vi "ApproachMonitor.vi"() -> ()   [LabVIEW 2021]
uses:
  <userlib>/Nanonis Prog Interface V5/Nanonis Prog Interface.lvlib
panel:
  in  "Walker Frequency (Hz)":dbl=220.0
  in  "Bias (V)":dbl=-1.2 format="%#_6p"
  in  "Walker voltage (V)":dbl=220.0
  in  "Time between checks (ms)":i32=20000
  in  "Averages":i32=50
  in  "milliseconds to wait":u32=1000
  out "Delta":cluster{i32, sgl}[](graph)
  out "Capacitance":cluster{i32, sgl}[](graph)
  # "MAKE SURE FAST APPROACH IS NOT TURNED ON!!!!!!!!!!"
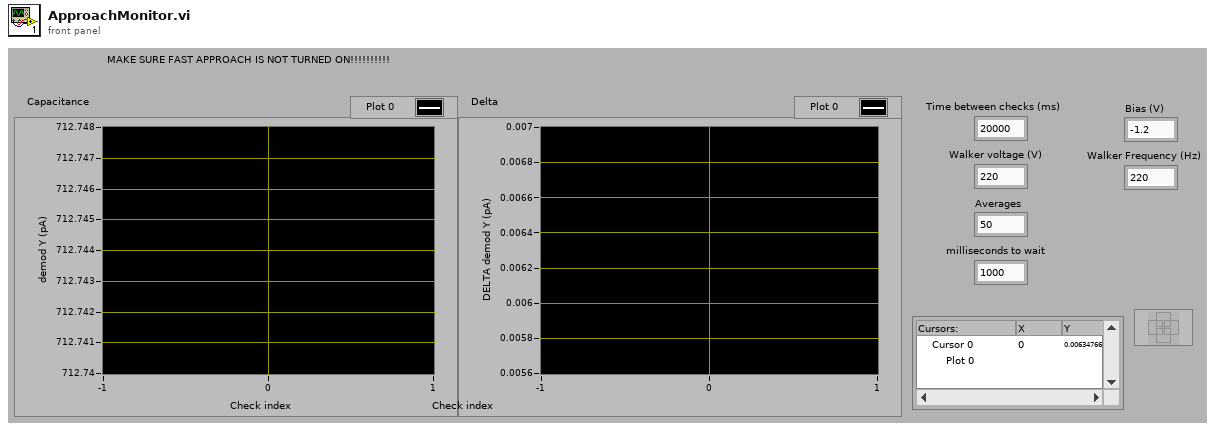
[diagram p1: front panel]
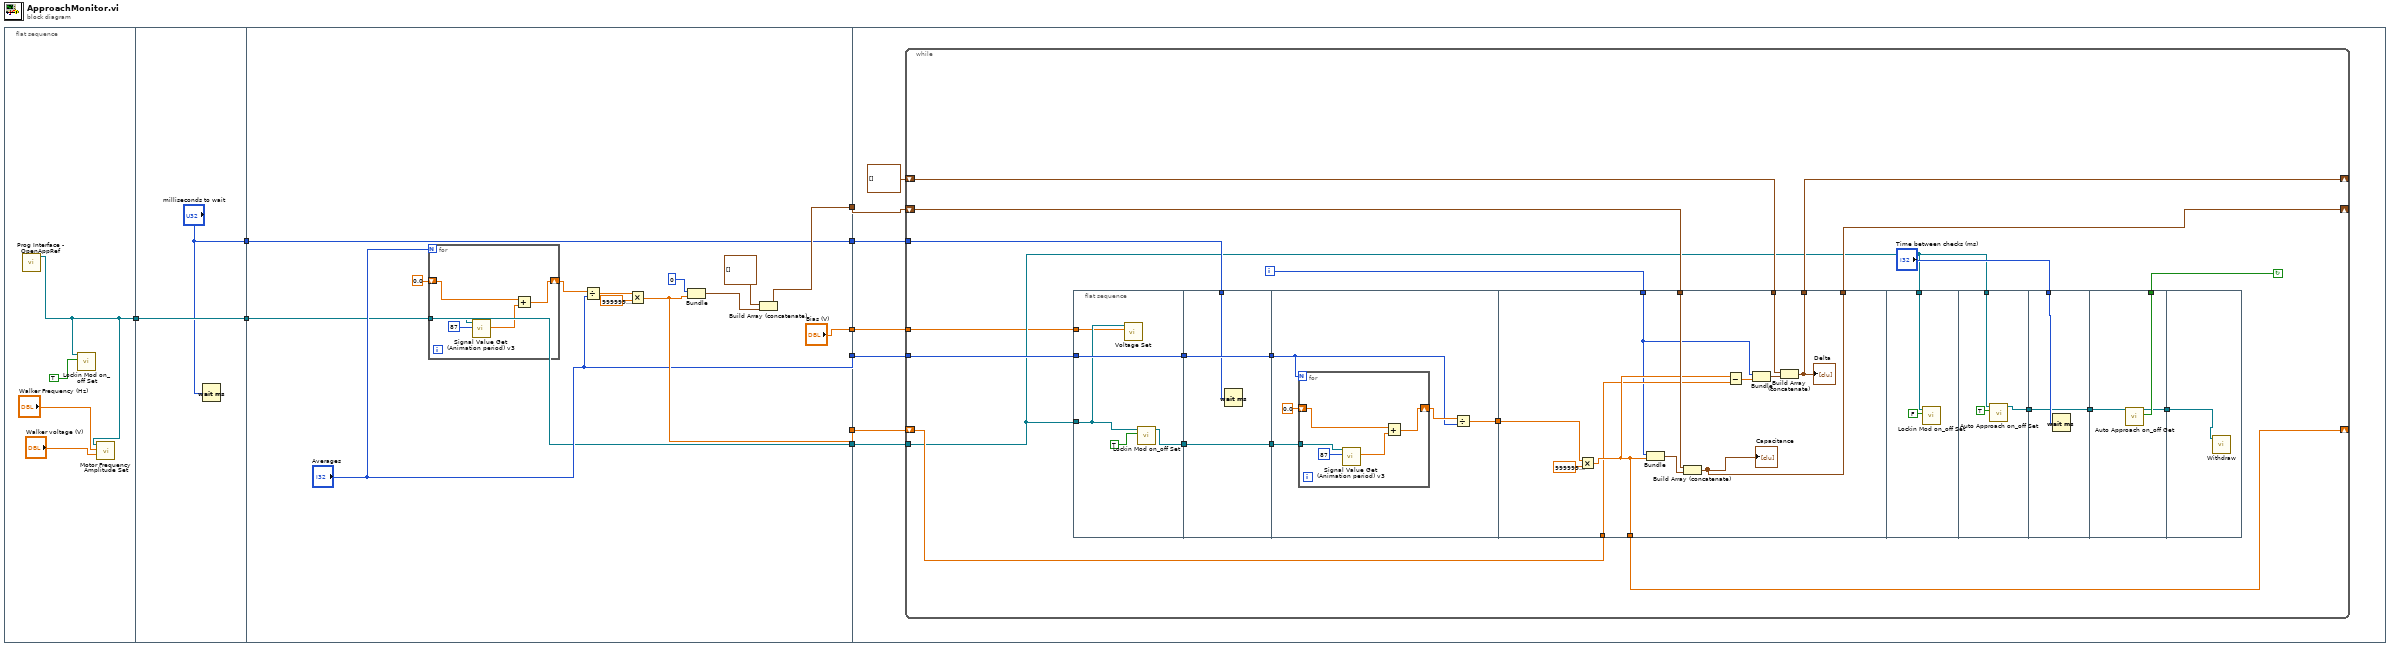
[diagram p0: block diagram]
diagram:
  n1 = flat-sequence {
    tunnel: [w11] -> w4
    tunnel: w4 -> [w15]
    tunnel: [w15] -> w3
    tunnel: ["milliseconds to wait"] -> w2
    tunnel: ["Averages"] -> w9
    tunnel: [w21] -> w8
    tunnel: [w24] -> w7
    tunnel: [w23] -> w6
    tunnel: w3 -> [w21]
    tunnel: [w20] -> w5
    tunnel: w2 -> [w20]
    tunnel: ["Bias (V)"] -> w1
    tunnel: w9 -> [w40]
    tunnel: w8 -> [w39]
    tunnel: w7 -> [w38]
    tunnel: w6 -> [w37]
    tunnel: w5 -> [w35]
    tunnel: w1 -> [w34]
    frame #0 {
      n2 = call <userlib>:"Prog Interface - OpenAppRef.vi"() -> ("Application reference"=w11:refnum<vi>)  [unwired: 6 in, 1 out]
      n3 = call <userlib>:"Lockin Mod on_off Set.vi"("Lockin ON/OFF"=TRUE, "Application ref in"=w11) -> ()  [unwired: 8 in, 2 out]
      n4 = call <userlib>:"Motor Frequency Amplitude Set.vi"("Amplitude (V) (NaN=no change)"="Walker voltage (V)", "Frequency (Hz) (NaN=no change)"="Walker Frequency (Hz)", "Application ref in"=w11) -> ()  [unwired: 7 in, 2 out]
    }
    frame #1 {
      n5 = Wait (ms)(milliseconds to wait="milliseconds to wait") -> ()  [unwired: 1 out]
    }
    frame #2 {
      n6 = for {
        N: "Averages" -> [_]
        shift-right: [w31] -> w27
        shift-left: sgl 0.0 ("Signal value") -> [w30]
        tunnel: w21 -> [w29]
        n7 = call <userlib>:"Signal Value Get (Animation period) v3.vi"("Signal index (0-127)"=i8 87, "Application ref in"=w29) -> ("Signal value"=w32:sgl)  [unwired: 6 in, 2 out]
        n8 = Add(x=w30, y=w32) -> (x+y=w31:sgl)
      }
      n9 = Divide(x=w27, y="Averages") -> (x/y=w28:sgl)
      n10 = Multiply(x=w28, y=sgl 1000000000000.0) -> (x*y=w23:sgl)
      n11 = Bundle(0, w23) -> (w18:cluster{i32, sgl})  [unwired: 1 in]
      n12 = Build Array (concatenate)(cluster{i32, sgl}[] [], w18) -> (w24:cluster{i32, sgl}[])
    }
    frame #3 {
      n13 = while {
        shift-right: [w60] -> _
        shift-left: w38 -> [w57]
        shift-right: [w59] -> _
        shift-left: cluster{i32, sgl}[] [] -> [w56]
        shift-right: [w55] -> _
        shift-left: w37 -> [w54]
        tunnel: w40 -> [w58]
        tunnel: w39 -> [w43]
        tunnel: w35 -> [w44]
        tunnel: w34 -> [w41]
        i -> [w49]
        stop <- w42 continue-if-true
        n14 = flat-sequence {
          tunnel: w43 -> [w63]
          tunnel: w58 -> [w66]
          tunnel: [w66] -> w48
          tunnel: [w65] -> w46
          tunnel: w41 -> [w62]
          tunnel: w48 -> [w69]
          tunnel: [w69] -> w47
          tunnel: w46 -> [w68]
          tunnel: [w68] -> w45
          tunnel: w44 -> [w67]
          tunnel: [w72] -> w61
          tunnel: w47 -> [w71]
          tunnel: w45 -> [w70]
          tunnel: w61 -> [w89]
          tunnel: [w87] -> w60
          tunnel: [w88] -> w59
          tunnel: w57 -> [w86]
          tunnel: w56 -> [w85]
          tunnel: [w84] -> w55
          tunnel: w54 -> [w83]
          tunnel: w49 -> [w82]
          tunnel: w43 -> [w92]
          tunnel: w43 -> [w95]
          tunnel: [w94] -> w51
          tunnel: "Time between checks (ms)" -> [w98]
          tunnel: [w97] -> w52
          tunnel: w51 -> [w97]
          tunnel: [w101] -> w42
          tunnel: w52 -> [w100]
          tunnel: [w99] -> w50
          tunnel: w50 -> [w102]
          frame #0 {
            n15 = call <userlib>:"Voltage Set.vi"("Bias (V)"=w62, "Application ref in"=w63) -> ()  [unwired: 8 in, 2 out]
            n16 = call <userlib>:"Lockin Mod on_off Set.vi"("Lockin ON/OFF"=TRUE, "Application ref in"=w63) -> ("Application ref out"=w65:refnum<vi>)  [unwired: 8 in, 1 out]
          }
          frame #1 {
            n17 = Wait (ms)(milliseconds to wait=w67) -> ()  [unwired: 1 out]
          }
          frame #2 {
            n18 = for {
              N: w71 -> [_]
              shift-right: [w77] -> w73
              shift-left: sgl 0.0 ("Signal value") -> [w76]
              tunnel: w70 -> [w75]
              n19 = call <userlib>:"Signal Value Get (Animation period) v3.vi"("Signal index (0-127)"=i8 87, "Application ref in"=w75) -> ("Signal value"=w78:sgl)  [unwired: 6 in, 2 out]
              n20 = Add(x=w76, y=w78) -> (x+y=w77:sgl)
            }
            n21 = Divide(x=w73, y=w71) -> (x/y=w72:sgl)
          }
          frame #3 {
            n22 = Multiply(x=w89, y=sgl 1000000000000.0) -> (x*y=w84:sgl)
            n23 = Bundle(w82, w84) -> (w80:cluster{i32, sgl})  [unwired: 1 in]
            n24 = Build Array (concatenate)(w86, w80) -> (w87:cluster{i32, sgl}[])
            "Capacitance" <- w87
            n25 = Subtract(x=w84, y=w83) -> (x-y=w91:sgl)
            n26 = Bundle(w82, w91) -> (w81:cluster{i32, sgl})  [unwired: 1 in]
            n27 = Build Array (concatenate)(w85, w81) -> (w88:cluster{i32, sgl}[])
            "Delta" <- w88
          }
          frame #4 {
            n28 = call <userlib>:"Lockin Mod on_off Set.vi"("Lockin ON/OFF"=FALSE, "Application ref in"=w92) -> ()  [unwired: 8 in, 2 out]
          }
          frame #5 {
            n29 = call <userlib>:"Auto Approach on_off Set.vi"("Auto approach start/stop (F)"=TRUE, "Application ref in"=w95) -> ("Application ref out"=w94:refnum<vi>)  [unwired: 6 in, 1 out]
          }
          frame #6 {
            n30 = Wait (ms)(milliseconds to wait=w98) -> ()  [unwired: 1 out]
          }
          frame #7 {
            n31 = call <userlib>:"Auto Approach on_off Get.vi"("Application ref in"=w100) -> ("Auto approach on/off status"=w101:bool, "Application ref out"=w99:refnum<vi>)  [unwired: 6 in, 1 out]
          }
          frame #8 {
            n32 = call <userlib>:"Withdraw.vi"("Application ref in"=w102) -> ()  [unwired: 9 in, 2 out]
          }
        }
      }
    }
  }
